vi "cursor_next.vi"(8 "error in (no error)":errorcluster, 9 "ms wait (-1)":i32=-1, 11 "cursor in":T1) -> (0 "error out":errorcluster, 1 "timed out?":bool, 2 "object":variant, 3 "cursor out":T1, 5 "object count":i32)   [LabVIEW 2017, in "rethinkdb.lvlib"]
uses:
  rethinkdb.lvlib
  cursor_refnum.ctl
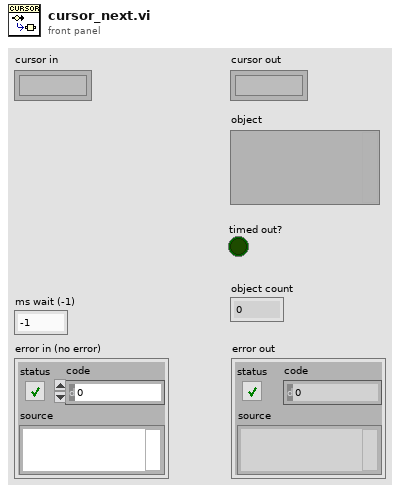
[diagram p1: front panel]
types:
  T1 = typedef "rethinkdb.lvlib/cursor_refnum.ctl" = refnum<k1>
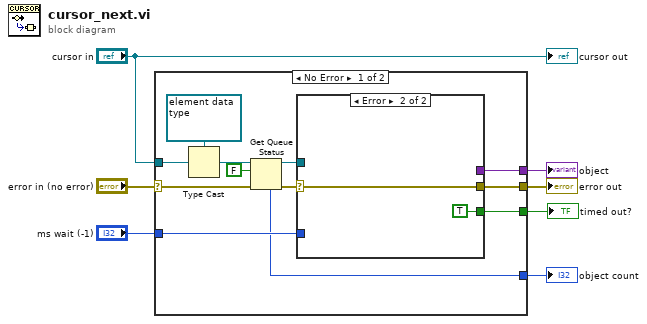
[diagram p0: block diagram]
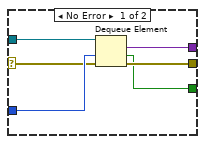
[diagram p2: hidden frame]
diagram:
  n1 = case shown="No Error" "error in (no error)" {
    selector: "error in (no error)" -> [w16 w28]
    tunnel: "ms wait (-1)" -> [w17 _]
    tunnel: "cursor in" -> [w19 _]
    tunnel: [w13 w28] -> w5
    tunnel: [w12 _] -> w3
    tunnel: [w14 _] -> w2
    tunnel: [w8 _] -> w1
    frame No Error {
      n2 = Type Cast(type=refnum<queue> refnum ("queue out"), x=w19) -> (*(type *) &x=w11:refnum<queue>)
      n3 = Get Queue Status(queue=w11, return elements? (F)=FALSE, error in (no error)=w16) -> (queue out=w10:refnum<queue>, error out=w9:errorcluster, # elements in queue=w12:i32)  [unwired: 5 out]
      n4 = case shown="Error" w9 {
        selector: w9 -> [w21 w27]
        tunnel: w17 -> [w25 _]
        tunnel: w10 -> [w24 _]
        tunnel: [w23 _] -> w14
        tunnel: [w22 w27] -> w13
        tunnel: [w20 TRUE ("timed out?")] -> w8
        frame No Error {
          n5 = Dequeue Element(queue=w24, timeout in ms (-1)=w25, error in (no error)=w21) -> (element=w23:variant, timed out?=w20:bool, error out=w22:errorcluster)  [unwired: 1 out]
        }
        frame Error {
        }
      }
    }
    frame Error {
    }
  }
  "error out" <- w5
  "object" <- w2
  "object count" <- w3
  "timed out?" <- w1
  "cursor out" <- "cursor in"
